vi "compound.vi"(1 "In Array":u16[](array[numeric])) -> (0 "Result":u32[](array[numeric]))   [LabVIEW 2015]
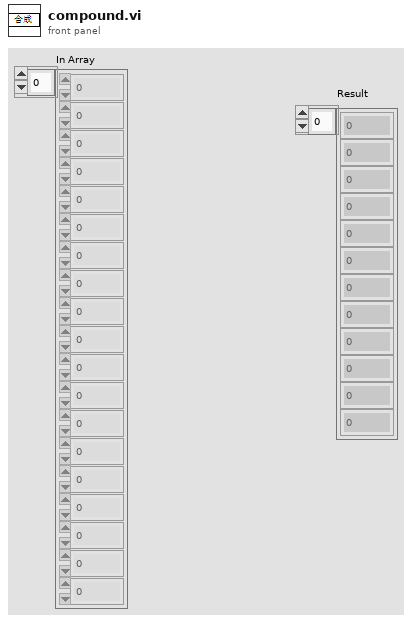
[diagram p1: front panel]
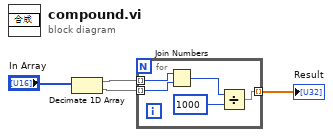
[diagram p0: block diagram]
diagram:
  n1 = Decimate 1D Array("In Array") -> (w2:u16[], w1:u16[])
  n2 = for {
    tunnel: w2 -> [w9] mode=indexing
    tunnel: w1 -> [w8] mode=indexing
    tunnel: [w5] -> w4 mode=indexing
    n3 = Join Numbers(hi=w9, lo=w8) -> ((hi.lo)=w7:u32)
    n4 = Divide(x=w7, y=u32 1000) -> (x/y=w5:dbl)
  }
  "Result" <- w4
